vi "gp-env.vi"() -> ()   [LabVIEW 2020, in "GPackTools.lvlib"]
uses:
  GPackTools.lvlib
panel:
  out "Not on Path":bool
  # "Configuring the system to use GPack..."
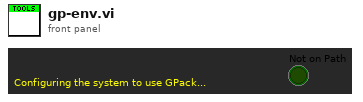
[diagram p1: front panel]
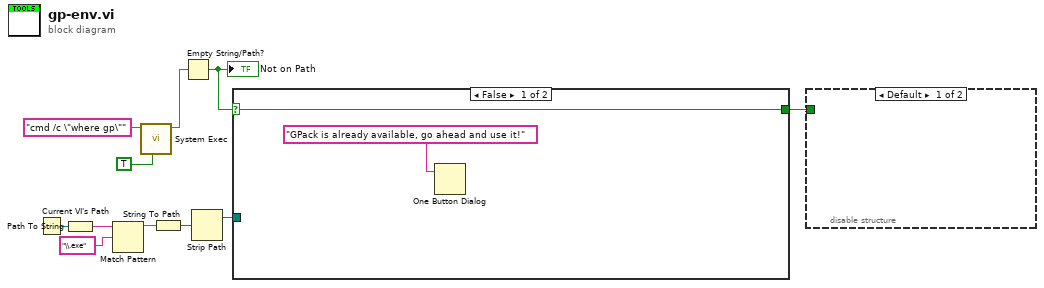
[diagram p0: block diagram]
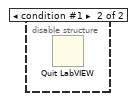
[diagram p2: hidden frame]
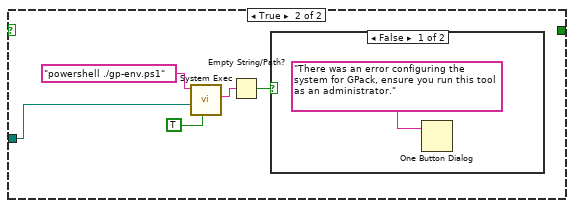
[diagram p3: hidden frame]
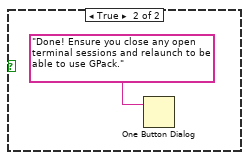
[diagram p4: hidden frame]
diagram:
  n1 = Current VI's Path() -> (path=w4:path)
  n2 = Path To String(path=w4) -> (string=w5:string)
  n3 = Match Pattern(string=w5, regular expression="\\.exe") -> (before substring=w6:string)  [unwired: 1 in, 3 out]
  n4 = call <vilib>:"System Exec.vi"("run minimized? (F)"=TRUE, "command line"="cmd /c \"where gp\"") -> ("standard output"=w9:string)  [unwired: 6 in, 3 out]
  n5 = String To Path(string=w6) -> (path=w7:path)
  n6 = Empty String/Path?(string/path=w9) -> (empty?=w8:bool)
  "Not on Path" <- w8
  n7 = Strip Path(path=w7) -> (stripped path=w2:path)  [unwired: 1 out]
  n8 = case shown="False" w8 {
    selector: w8 -> [w12 _]
    tunnel: w2 -> [_ w17]
    tunnel: [w12 _] -> w1
    frame False {
      n9 = One Button Dialog(message="GPack is already available, go ahead and use it!") -> ()  [unwired: 1 in, 1 out]
    }
    frame True {
      n10 = call <vilib>:"System Exec.vi"("run minimized? (F)"=TRUE, "working directory"=w17, "command line"="powershell ./gp-env.ps1") -> ("standard error"=w16:string)  [unwired: 5 in, 3 out]
      n11 = Empty String/Path?(string/path=w16) -> (empty?=w15:bool)
      n12 = case shown="False" w15 {
        frame False {
          n13 = One Button Dialog(message="There was an error configuring the system for GPack, ensure you run this tool as an administrator.") -> ()  [unwired: 1 in, 1 out]
        }
        frame True {
          n14 = One Button Dialog(message="Done! Ensure you close any open terminal sessions and relaunch to be able to use GPack.") -> ()  [unwired: 1 in, 1 out]
        }
      }
    }
  }
  n15 = disable-structure shown="Default" {
    disable-tunnel: w1 -> [_ _]
    frame condition #0 (active) {
    }
    frame condition #1 {
      n16 = Quit LabVIEW() -> ()  [unwired: 1 in]
    }
  }
